vi "Max Read Array.vi"(8 "error in":errorcluster, 11 "Max Current Limit in":refnum<class "Current Limit.lvclass">) -> (0 "error out":errorcluster, 1 "Changed or First Call?":bool, 2 "Current Max SP Limit":dbl[](array[numeric]), 3 "Max Current Limit out":refnum<class "Current Limit.lvclass">)   [LabVIEW 2023, in "Current Limit.lvclass"]
uses:
  Current Limit.lvclass
  Parents/Limit/Limit.lvclass
  Current Limit.lvclass/Current Limit.ctl
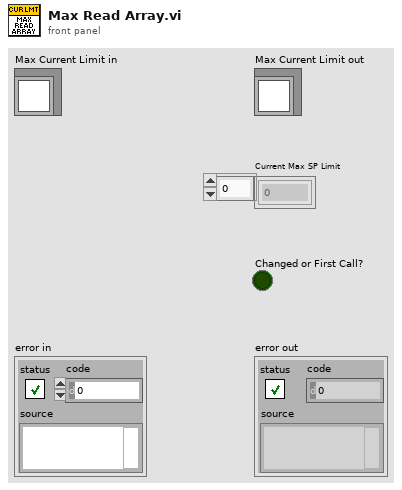
[diagram p1: front panel]
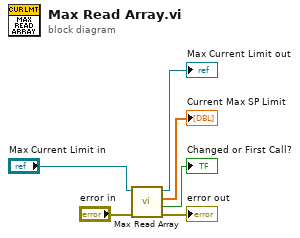
[diagram p0: block diagram]
diagram:
  n1 = call-parent "Max Read Array.vi"("error in"="error in", "Max Limit in"="Max Current Limit in") -> ("error out"=→"error out":errorcluster, "Changed or First Call?"=→"Changed or First Call?":bool, "Current Max Limit"=→"Current Max SP Limit":dbl[], "Max Limit out"=→"Max Current Limit out":refnum<class "Current Limit.lvclass">)  [unwired: 6 in]
